vi "Test Generate Mock Class Inherits from Mock.vi"(8 "error in (no error)":errorcluster, 11 "Test Case In":refnum<class "Pure Mock Class Generator Test.lvclass">) -> (0 "error out":errorcluster, 3 "Test Case Out":refnum<class "Pure Mock Class Generator Test.lvclass">)   [LabVIEW 2020, in "Pure Mock Class Generator Test.lvclass"]
uses:
  Pure Mock Class Generator Test.lvclass
  C:/Program Files (x86)/National Instruments/LabVIEW 2020/vi.lib/Astemes/LUnit/Test Case.lvclass
  <vilib>/Astemes/LUnit/Test Case.lvclass/Test Case.ctl
  d61b9b24-4b0f-44ef-a9bb-4996cb077d5f.vi
  <vilib>/Astemes/LUnit/Append Pass Result.vi
  <vilib>/Astemes/LUnit/Append Fail Result.vi
  <vilib>/Astemes/LUnit/Describe Comparison.vi
  <vilib>/Astemes/LUnit/Compare Variants.vi
  <vilib>/Astemes/LUnit/Variant to string.vi
  <vilib>/Utility/Data Type/Get Type Information.vi
  <vilib>/Utility/LVClass/Get LV Class Name.vi
  source/Scripting/Pure Mock Class Generator/Pure Mock Class Generator.lvclass
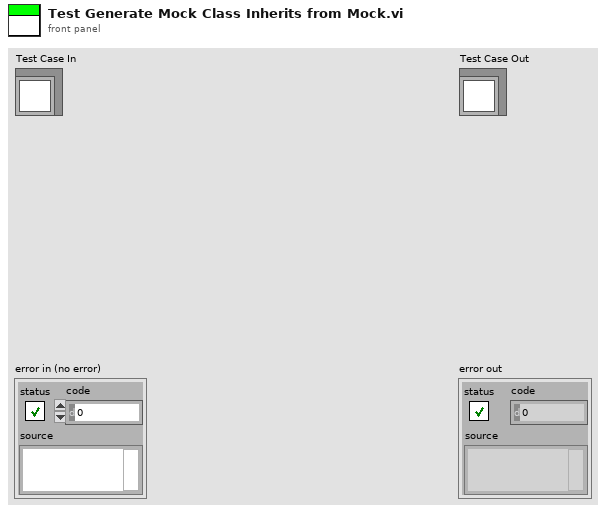
[diagram p1: front panel]
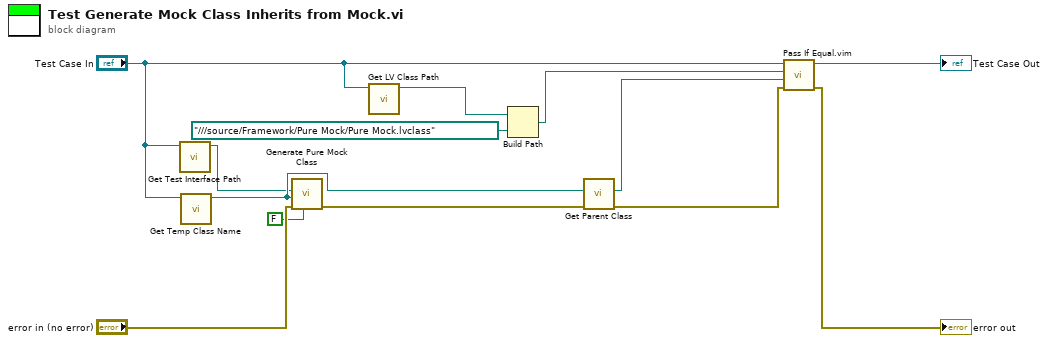
[diagram p0: block diagram]
diagram:
  n1 = call "Get Test Interface Path.vi"("Mock Class Generator Test in"="Test Case In") -> ("Test Class Path"=w6:path)  [unwired: 10 in]
  n2 = call "Get Temp Class Name.vi"("Mock Class Generator Test in"="Test Case In") -> ("Test Class Path"=w10:path)  [unwired: 10 in]
  n3 = call "Generate Pure Mock Class.vi"("Add to lvproj?"=FALSE, "error in (no error)"="error in (no error)", "Destination Class Path"=w10, "Source Class Path"=w6) -> ("error out"=w9:errorcluster)  [unwired: 7 in]
  n4 = call <vilib>:"Get LV Class Path.vi"("object"="Test Case In") -> ("class path"=w3:path)  [unwired: 9 in, 1 out]
  n5 = Build Path(base path=w3, name or relative path=path "../../../source/Framework/Pure Mock/Pure Mock.lvclass") -> (appended path=w1:path)
  n6 = call "Get Parent Class.vi"("error in (no error)"=w9, "Test Class Path"=w10) -> ("error out"=w8:errorcluster, "Path"=w7:path)  [unwired: 8 in]
  n7 = call "Pass If Equal.vim"("error in (no error)"=w8, "Actual"=w7, "Expected"=w1, "LUnit Test Case In"="Test Case In") -> ("error out"=→"error out":errorcluster, "LUnit Test Case Out"=→"Test Case Out":refnum<class "Pure Mock Class Generator Test.lvclass">)  [unwired: 6 in]
